vi "Untitled 1.vi"() -> ()   [LabVIEW 2015]
uses:
  <vilib>/Math Plots/2D Math Plots/2D Compass/2D Compass XCtrl/2D Compass.xctl
  <vilib>/Math Plots/2D Math Plots/2D Compass/2D Compass Datatype/Public/Plot Helper (Vector).vi
  <vilib>/Math Plots/2D Math Plots/2D Compass/2D Compass Datatype/Public/Plot Helper (Complex).vi
  <vilib>/Math Plots/2D Math Plots/2D Compass/2D Compass Datatype/2D Compass Datatype.lvclass
panel:
  out "2D Compass 2":refnum<class "2D Plot Datatype.lvclass">[](xcontrol)
  in  "Array":cdb[](array[numeric])
  in  "Numeric Control":i32
  in  "stepsize":i32
  in  "Stop Button":bool
  out "2D Compass":refnum<class "2D Plot Datatype.lvclass">[](xcontrol)
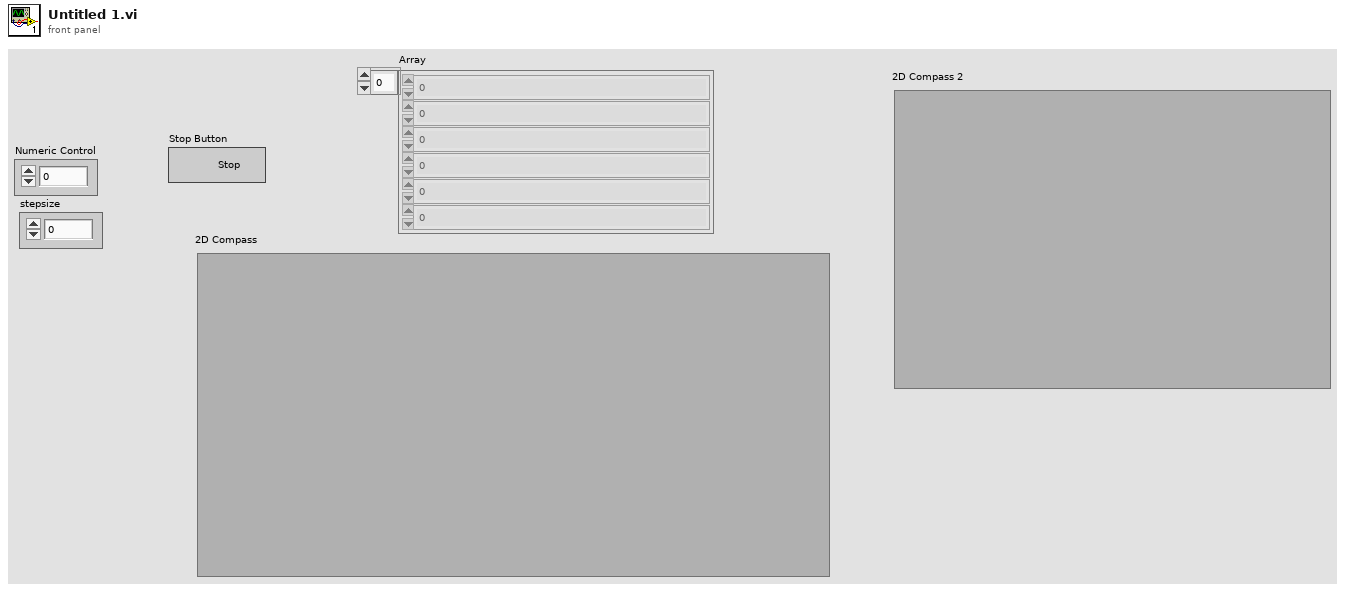
[diagram p1: front panel]
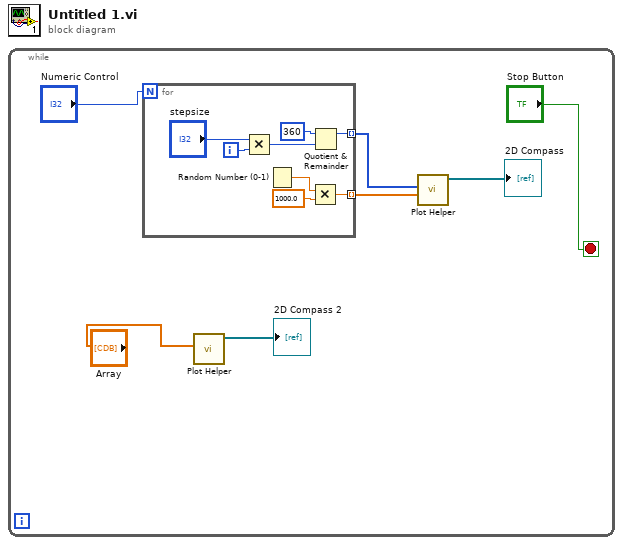
[diagram p0: block diagram]
diagram:
  n1 = while {
    stop <- "Stop Button" stop-if-true
    n2 = for {
      N: "Numeric Control" -> [_]
      tunnel: [w14] -> w6 mode=indexing
      tunnel: [w10] -> w5 mode=indexing
      i -> [w9]
      n3 = Multiply(x="stepsize", y=w9) -> (x*y=w12:i32)
      n4 = Random Number (0-1)() -> (number: 0 to 1=w8:dbl)
      n5 = Multiply(x=w8, y=1000.0) -> (x*y=w14:dbl)
      n6 = Quotient & Remainder(x=360, y=w12) -> (x-y*floor(x/y)=w10:i32)  [unwired: 1 out]
    }
    n7 = call-poly <vilib>:"Plot Helper.vi"("z vector"="Array") -> ("2D Plot Class Obj Array out"=→"2D Compass 2":refnum<class "2D Plot Datatype.lvclass">[])  [unwired: 2 in, 8 out]
    n8 = call-poly <vilib>:"Plot Helper.vi"("radius vector"=w6, "theta vector"=w5) -> ("2D Plot Class Obj Array out"=→"2D Compass":refnum<class "2D Plot Datatype.lvclass">[])  [unwired: 2 in, 7 out]
  }
